vi "CommunicationActivity.vi"() -> ()   [LabVIEW 2013]
panel:
  in  "CommunicationActivity":T1
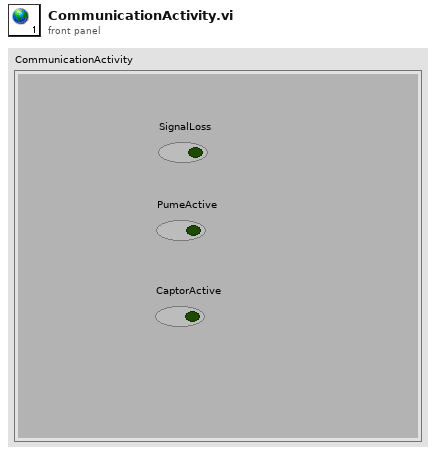
[diagram p1: front panel]
types:
  T1 = cluster{"SignalLoss":bool, "PumeActive":bool, "CaptorActive":bool}
diagram:
